vi "Get SMO Name from Error Event.vi"(8 "error in (no error)":errorcluster, 9 "Error":refnum<user-event>, 10 "SMOs":refnum<class "SMO.lvclass">[](array[class])) -> (0 "error out":errorcluster, 2 "class:SMO name":string)   [LabVIEW 2019, in "Logger.Error.lvclass"]
uses:
  Logger.Error.lvclass
  <vilib>/JKI/JKI SMO/SMO/SMO.lvclass
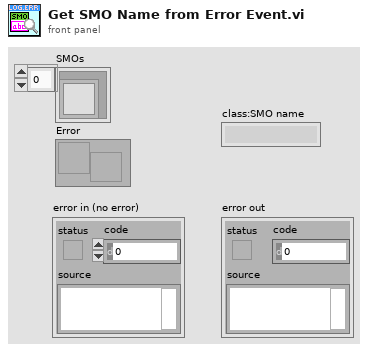
[diagram p1: front panel]
types:
  T1 = typedef "SMO.lvclass/Public Events.ctl" = cluster{"Error":refnum<user-event>, "State":refnum<user-event>, "Reserve State":refnum<user-event>}
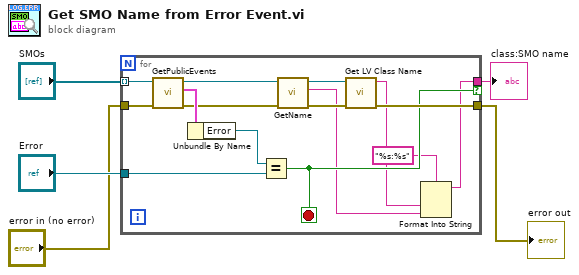
[diagram p0: block diagram]
diagram:
  n1 = for {
    tunnel: "SMOs" -> [w20] mode=indexing
    tunnel: "Error" -> [w17]
    tunnel: [w7] -> w1 if=w10
    tunnel: "error in (no error)" -> [w12]
    tunnel: [w11] -> w2
    stop <- w10 stop-if-true
    n2 = call <vilib>:"GetPublicEvents.vi"("error in (no error)"=w12, "SMO"=w20) -> ("error out"=w16:errorcluster, "Public Events"=w19:T1, "SMO out"=w15:refnum<class "SMO.lvclass">)  [unwired: 7 in]
    n3 = Unbundle By Name(w19) -> ("Error"=w18:refnum<user-event>)
    n4 = Equal?(x=w18, y=w17) -> (x = y?=w10:bool)
    n5 = call <vilib>:"GetName.vi"("error in (no error)"=w16, "SMO"=w15) -> ("error out"=w13:errorcluster, "Name"=w8:string, "SMO out"=w14:refnum<class "SMO.lvclass">)  [unwired: 6 in, 1 out]
    n6 = call <vilib>:"Get LV Class Name.vi"("error in (no error)"=w13, "object"=w14) -> ("error out"=w11:errorcluster, "class name"=w6:string)  [unwired: 8 in]
    n7 = Format Into String(format string="%s:%s", w6, w8) -> (resulting string=w7:string)  [unwired: 2 in, 1 out]
  }
  "error out" <- w2
  "class:SMO name" <- w1
